vi "booleo-case structure(1).vi"() -> ()   [LabVIEW 2013]
panel:
  out "Status":bool
  out "Result":string
  in  "Motor Control":bool
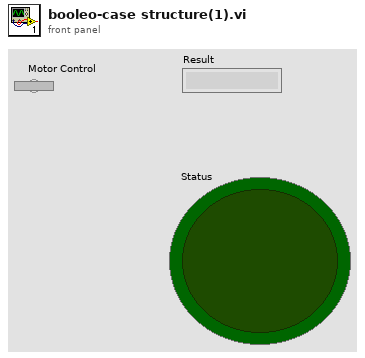
[diagram p1: front panel]
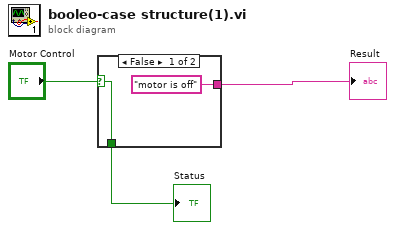
[diagram p0: block diagram]
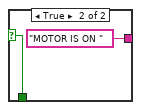
[diagram p2: hidden frame]
diagram:
  n1 = case shown="False" "Motor Control" {
    selector: "Motor Control" -> [w4 w6]
    tunnel: ["motor is off" ("String") "MOTOR IS ON " ("String")] -> w2
    tunnel: [w4 w6] -> w1
    frame False {
    }
    frame True {
    }
  }
  "Result" <- w2
  "Status" <- w1
